vi "init arduino.vi"(11 "VISA Refnum in":refnum<visa-resource-name>) -> (0 "error out":errorcluster, 3 "Arduino Resource":T1)   [LabVIEW 2016]
uses:
  <vilib>/LabVIEW Interface for Arduino/Type Defs/Arduino Resource.ctl
  <vilib>/LabVIEW Interface for Arduino/Type Defs/Board Type.ctl
  <vilib>/LabVIEW Interface for Arduino/Type Defs/Pin Mode.ctl
  <vilib>/LabVIEW Interface for Arduino/LabVIEW Interface for Arduino.lvlib
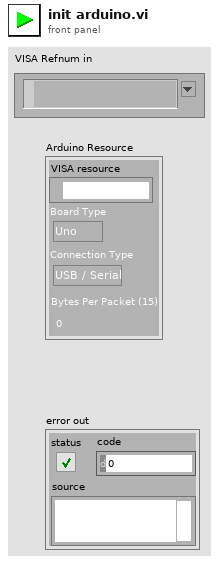
[diagram p1: front panel]
types:
  T1 = typedef "LabVIEW Interface for Arduino.lvlib/Arduino Resource.ctl" = cluster{"VISA resource":refnum<visa-resource-name>, "Board Type":T2, "Connection Type":enum8{"USB / Serial"}, "Bytes Per Packet (15)":u8}
  T2 = typedef "LabVIEW Interface for Arduino.lvlib/Board Type.ctl" = enum16{"Uno", "Dimuelanove w/Atmega 328", "Mega 2560"}
  T3 = typedef "LabVIEW Interface for Arduino.lvlib/Pin Mode.ctl" = enum8{"Input", "Output"}
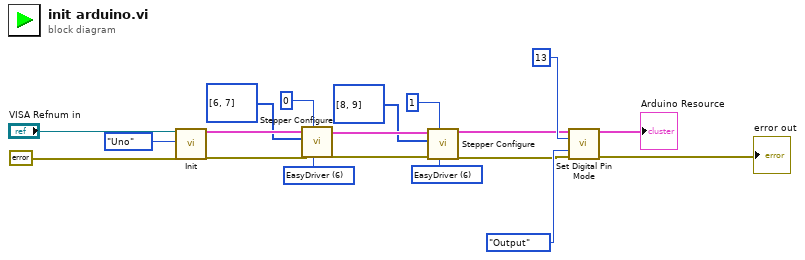
[diagram p0: block diagram]
diagram:
  w11 = u8 6 items=["2 Wire (Pulse & Direction)"=1, "2 Wire"=2, "4 Wire"=4, "EasyDriver"=6, "AF Motor Shield (Stepper 1 & 2 Only)"=5] ("Control Method")
  w12 = u8 6 items=["2 Wire (Pulse & Direction)"=1, "2 Wire"=2, "4 Wire"=4, "EasyDriver"=6, "AF Motor Shield (Stepper 1 & 2 Only)"=5] ("Control Method")
  n1 = call <vilib>:"Init.vi"("VISA resource"="VISA Refnum in", "Board Type (Uno)"=Board_Type."Uno", "error in"=errorcluster {"status"=FALSE, "code"=0, "source"=""}) -> ("Arduino Resource"=w9:T1, "error out"=w10:errorcluster)  [unwired: 15 in]
  n2 = call <vilib>:"Stepper Configure.vi"("Control Method"=w11, "Stepper #"=u8 0, "error in"=w10, "Stepper Pins"=u8[] [6, 7], "Arduino Resource"=w9) -> ("error out"=w7:errorcluster, "Arduino Resource Out"=w6:T1)  [unwired: 5 in]
  n3 = call <vilib>:"Stepper Configure.vi"("Control Method"=w12, "Stepper #"=u8 1, "error in"=w7, "Stepper Pins"=u8[] [8, 9], "Arduino Resource"=w6) -> ("error out"=w2:errorcluster, "Arduino Resource Out"=w1:T1)  [unwired: 5 in]
  n4 = call <vilib>:"Set Digital Pin Mode.vi"("Arduino Resource"=w1, "Digital I/O Pin"=u8 13, "Pin Mode (Input)"=Pin_Mode."Output", "error in"=w2) -> ("Arduino Resource"=→"Arduino Resource":T1, "error out"=→"error out":errorcluster)  [unwired: 10 in]
